vi "Calibrate.vi"(7 "error in (no error)":errorcluster, 10 "VISA resource name":refnum<visa-resource-name>) -> (0 "error out":errorcluster, 1 "output raw":dbl, 2 "output / s":dbl, 3 "VISA resource name out":refnum<visa-resource-name>)   [LabVIEW 2017, in "GP22_TDC_Arduinoed.lvlib"]
doc: "Calibrate the GP22 by comparing its readings to its internal clock. \n\nThis function is not needed unless running in high speed mode. \n\nAssuming that the internal clock is running at 4MHz, this function will update the value stored in Globals.vi and used by ConvertTimes.vi to interpret uncalibrated data. N.B. the drift of the high speed internal clock should be corrected for by using the \"High Speed Calibration\" subVI: this subVI corrects for the drift of the TDC with respect to the high speed clock. \n\nAlso returns a number respresenting the resolution of an uncalibrated LSB from the TDC in seconds.\n\nCompared to the HF calibration, this should be run more often as it drifts more and also takes less time to correct."
uses:
  GP22_TDC_Arduinoed.lvlib
  Globals.vi
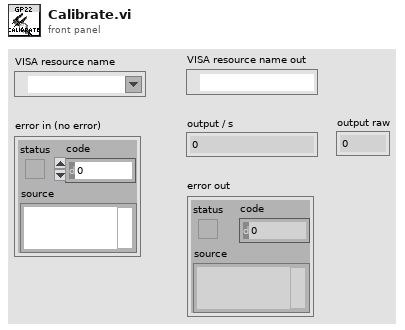
[diagram p1: front panel]
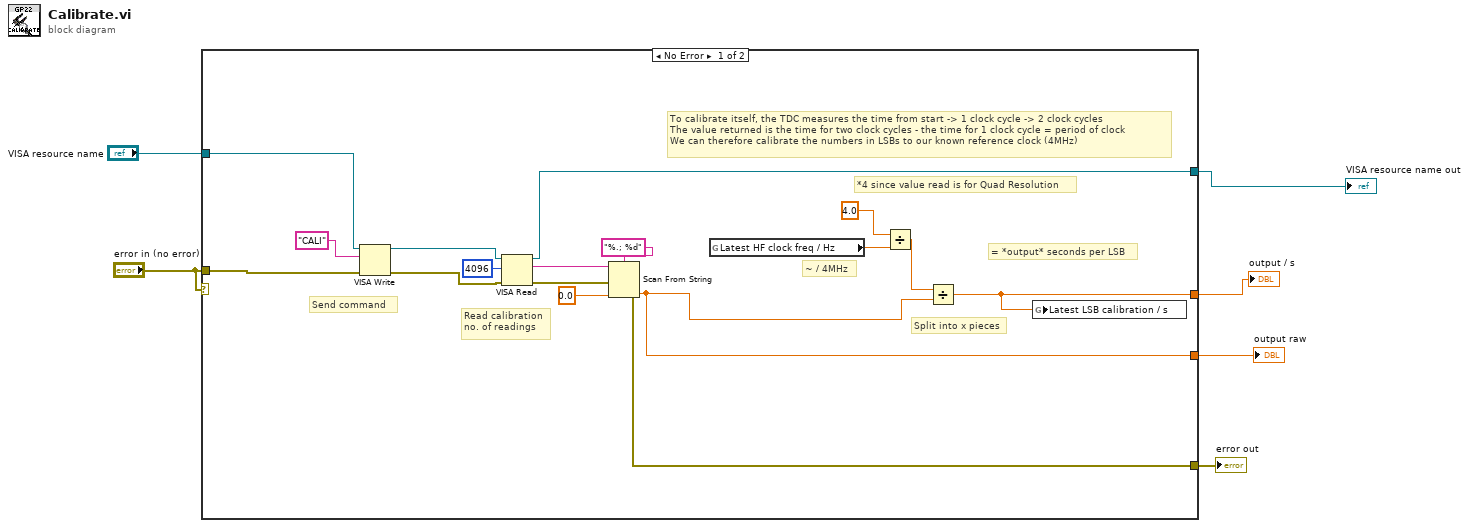
[diagram p0: block diagram]
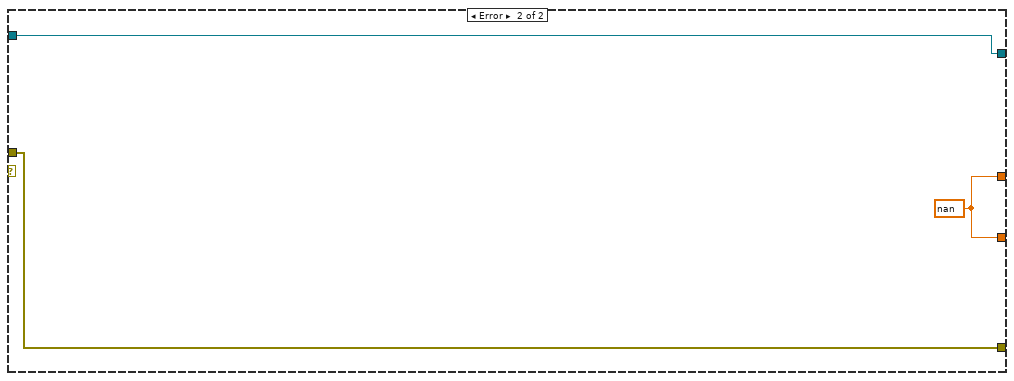
[diagram p2: hidden frame]
diagram:
  n1 = case shown="No Error" "error in (no error)" {
    tunnel: "error in (no error)" -> [w23 w26]
    tunnel: [w15 w26] -> w6
    tunnel: [w10 w24] -> w4
    tunnel: "VISA resource name" -> [w9 w24]
    tunnel: [w8 w25] -> w2
    tunnel: [w7 w25] -> w1
    frame No Error {
      # "To calibrate itself, the TDC measures the time from start -> 1 clock cycle -> 2 clock cycles\nThe value returned is the time for two clock cycles - the time for 1 clock cycle = period of clock\nWe can therefore calibrate the numbers in LSBs to our known reference clock (4MHz)"
      # "*4 since value read is for Quad Resolution"
      # "Read calibration\nno. of readings"
      # "Send command"
      # "= *output* seconds per LSB"
      # "Split into x pieces"
      # "~ / 4MHz"
      n2 = VISA Write(VISA resource name=w9, write buffer="CALI" ("command"), error in (no error)=w23) -> (VISA resource name out=w14:refnum<visa-resource-name>, error out=w22:errorcluster)  [unwired: 1 out]
      n3 = VISA Read(VISA resource name=w14, byte count=u32 4096, error in (no error)=w22) -> (VISA resource name out=w10:refnum<visa-resource-name>, read buffer=w19:string, error out=w17:errorcluster)  [unwired: 1 out]
      n4 = Scan From String(format string="%.; %d", input string=w19, error in=w17, default 1=0.0 ("default value 1")) -> (error out=w15:errorcluster, output 1=w7:dbl)  [unwired: 1 in, 2 out]
      n5 = global read "Globals.vi" "Latest HF clock freq / Hz"() -> (w11:dbl)
      n6 = Divide(x=4.0 ("y"), y=w11) -> (x/y=w12:dbl)
      n7 = Divide(x=w12, y=w7) -> (x/y=w8:dbl)
      n8 = global write "Globals.vi" "Latest LSB calibration / s"(w8) -> ()
    }
    frame Error {
      w25 = nan
    }
  }
  "error out" <- w6
  "VISA resource name out" <- w4
  "output / s" <- w2
  "output raw" <- w1
